vi "TSV_2_DSC.vi"(8 "error in (no error)":errorcluster, 10 "Enum":T1, 11 "path to txt file":path) -> (0 "error out":errorcluster)   [LabVIEW 2019, in "VCL_2_DSC.lvclass"]
uses:
  VCL_2_DSC.lvclass
  typedefs/write-enum.ctl
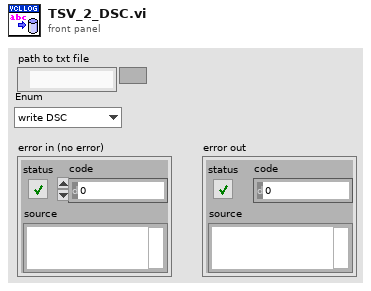
[diagram p1: front panel]
types:
  T1 = typedef "VCL_2_DSC.lvclass/write-enum.ctl" = enum16{"write DSC", "write TDMS", "no write"}
  T2 = typedef "VCL_2_DSC.lvclass/TSLtoLV-cluster.ctl" = cluster{"time name":string, "trace name":string, "time array":timestamp[], "trace array":dbl[]}
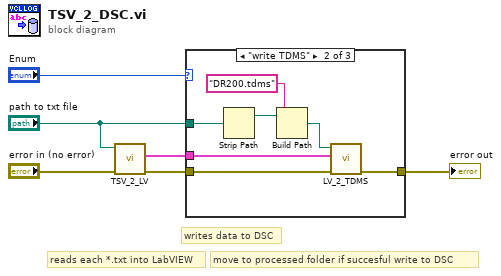
[diagram p0: block diagram]
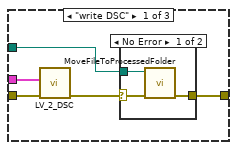
[diagram p2: hidden frame]
diagram:
  # "move to processed folder if succesful write to DSC"
  # "reads each *.txt into LabVIEW"
  # "writes data to DSC"
  n1 = call "TSV_2_LV.vi"("error in (no error)"="error in (no error)", "tsv file path (dialog if empty)"="path to txt file") -> ("error out"=w2:errorcluster, "data"=w3:T2[])  [unwired: 8 in]
  n2 = case shown="\"write TDMS\"" "Enum" {
    tunnel: w2 -> [w11 w22 w23]
    tunnel: w3 -> [w7 w21 _]
    tunnel: [w10 w20 w23] -> w4
    tunnel: "path to txt file" -> [w9 w19 _]
    frame "write DSC" {
      n3 = call "LV_2_DSC.vi"("error in (no error)"=w11, "data"=w7) -> ("error out"=w8:errorcluster)  [unwired: 9 in]
      n4 = case shown="No Error" w8 {
        selector: w8 -> [w12 w15]
        tunnel: [w14 w15] -> w10
        tunnel: w9 -> [w13 _]
        frame No Error {
          n5 = call "MoveFileToProcessedFolder.vi"("error in (no error)"=w12, "source file"=w13) -> ("error out"=w14:errorcluster)  [unwired: 8 in, 1 out]
        }
        frame Error {
        }
      }
    }
    frame "write TDMS" {
      n6 = Strip Path(path=w19) -> (stripped path=w18:path)  [unwired: 1 out]
      n7 = Build Path(base path=w18, name or relative path="DR200.tdms") -> (appended path=w16:path)
      n8 = call "LV_2_TDMS.vi"("error in (no error)"=w22, "data"=w21, "file path"=w16) -> ("error out"=w20:errorcluster)  [unwired: 8 in]
    }
    frame "no write", Default {
    }
  }
  "error out" <- w4
